vi "waitseq.vi"(8 "error in":errorcluster, 11 "time (ms)":u32) -> (0 "error out":errorcluster, 2 "millisecond timer value":u32, 3 "time out":u32)   [LabVIEW 2014]
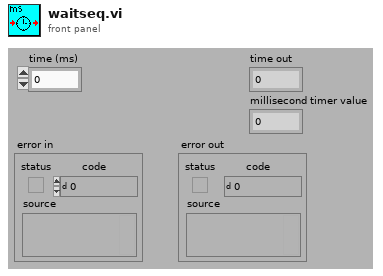
[diagram p1: front panel]
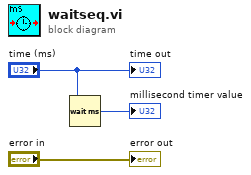
[diagram p0: block diagram]
diagram:
  n1 = Wait (ms)(milliseconds to wait="time (ms)") -> (millisecond timer value=→"millisecond timer value":u32)
  "error out" <- "error in"
  "time out" <- "time (ms)"
